vi "SaveDataSet.vi"(6 "AssetNodeMap":variant, 7 "do not write to database":bool, 8 "error in (no error)":errorcluster, 9 "Waveform":waveform(sgl), 10 "DataSetRegistry":T1, 11 "event in":T3) -> (0 "error out":errorcluster, 3 "event out":T3)   [LabVIEW 2017, in "CmsDataEventCreator.lvlib"]
uses:
  <vilib>/addons/InsightCM/Devices/Shared/Cms/CmsDataEventCreator/CmsDataEventCreator.lvlib
  <vilib>/addons/InsightCM/Devices/Shared/Common/DataEvent/controls/Event.ctl
  <vilib>/addons/InsightCM/MessageBus/Base/controls/DataEvent.ctl
  <vilib>/addons/InsightCM/MessageBus/Base/controls/KeyValuePair.ctl
  <vilib>/addons/InsightCM/Devices/Shared/Common/DataEvent/controls/DataSet.ctl
  <vilib>/addons/InsightCM/MessageBus/Base/controls/DataSetMetadata.ctl
  <vilib>/addons/InsightCM/MessageBus/Base/controls/TrendPoint.ctl
  <vilib>/addons/InsightCM/MessageBus/Base/controls/TrendAlarmUpdate.ctl
  <vilib>/addons/InsightCM/MessageBus/Base/controls/TrendAlarmTransition.ctl
  <vilib>/addons/InsightCM/Devices/Shared/Cms/CmsDataEventCreator/controls/DataSetRegistry.ctl
  <vilib>/addons/InsightCM/Devices/Shared/Common/DataEvent/controls/DataSetType.ctl
  <vilib>/addons/InsightCM/Devices/Shared/Common/DataEventCreator/DataEventCreator.lvlib
  <vilib>/addons/InsightCM/Utilities/PropertyHelpers/PropertyHelpers.lvlib
  <vilib>/addons/InsightCM/Devices/Shared/Common/DataEvent/DataEvent.lvlib
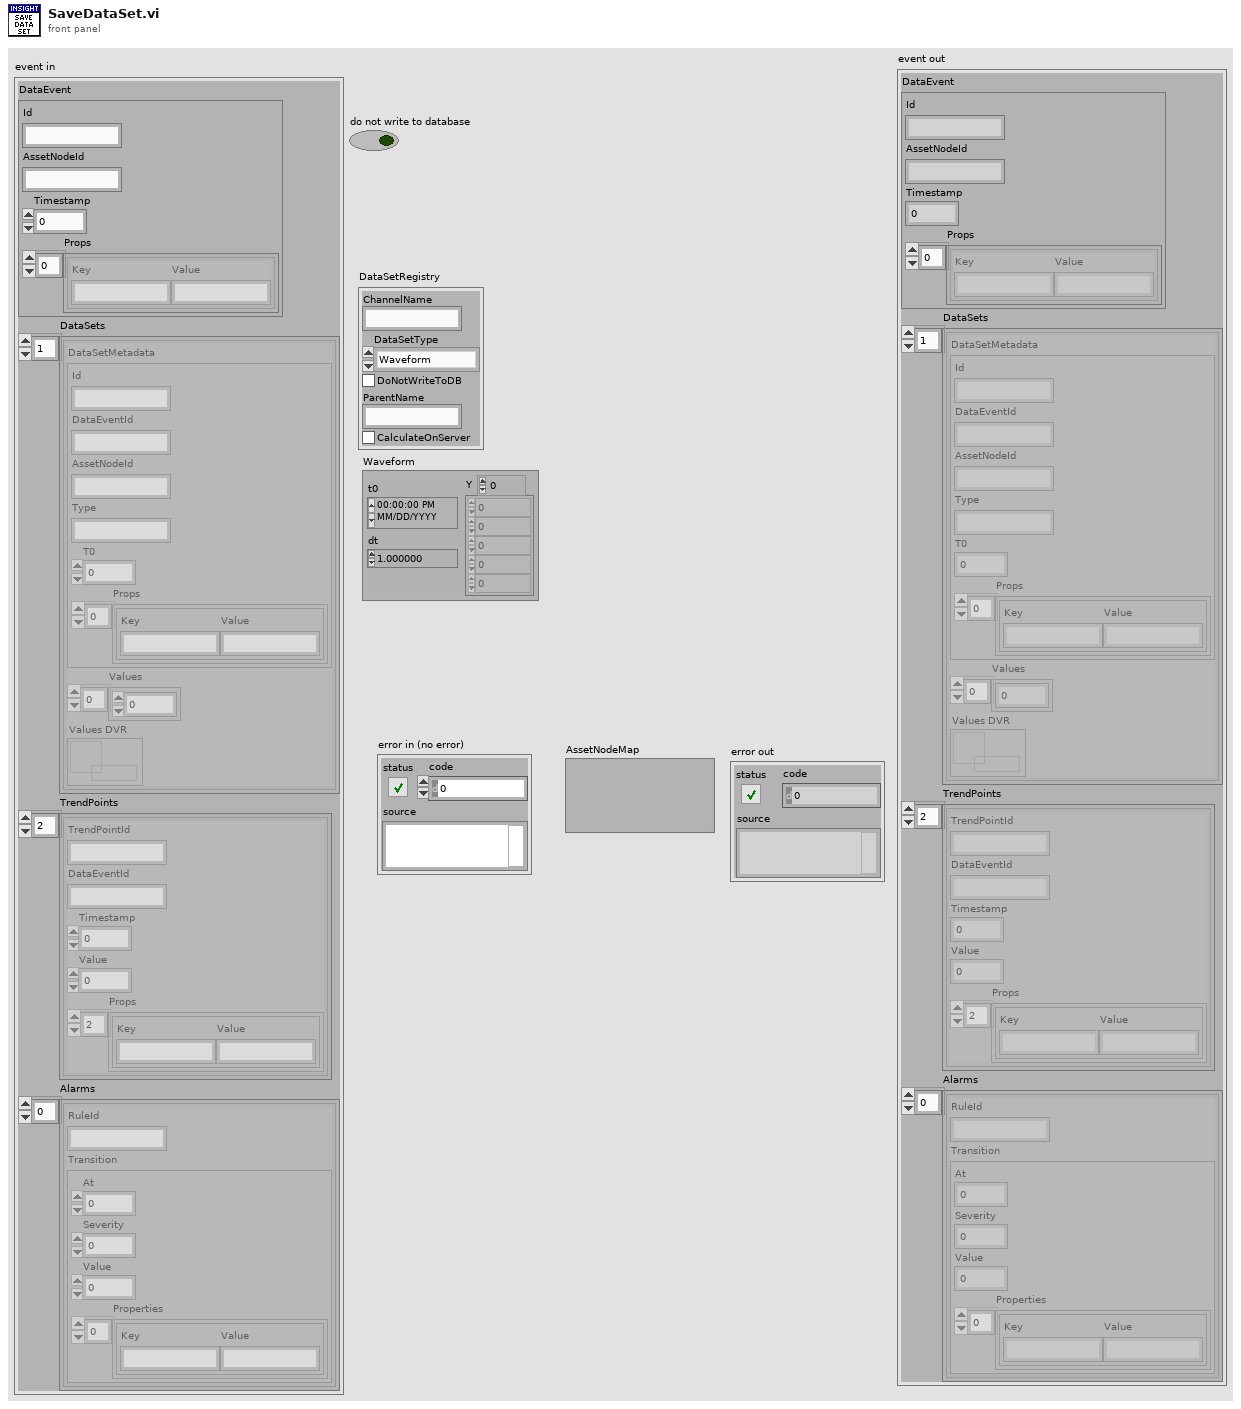
[diagram p1: front panel]
types:
  T1 = typedef "CmsDataEventCreator.lvlib/DataSetRegistry.ctl" = cluster{"ChannelName":string, "DataSetType":T2, "DoNotWriteToDB":bool, "ParentName":string, "CalculateOnServer":bool}
  T2 = typedef "DataEvent.lvlib/DataSetType.ctl" = enum16{"Waveform", "SpeedProfile", "ThermalImage", "EmsaSweep"}
  T3 = typedef "DataEvent.lvlib/Event.ctl" = cluster{"DataEvent":T4, "DataSets":T6[], "TrendPoints":T8[], "Alarms":T9[]}
  T4 = typedef "DataEvent.ctl" = cluster{"Id":string, "AssetNodeId":string, "Timestamp":i64, "Props":T5[]}
  T5 = typedef "KeyValuePair.ctl" = cluster{"Key":string, "Value":string}
  T6 = typedef "DataEvent.lvlib/DataSet.ctl" = cluster{"DataSetMetadata":T7, "Values":sgl[], "Values DVR":refnum<data-value>}
  T7 = typedef "DataSetMetadata.ctl" = cluster{"Id":string, "DataEventId":string, "AssetNodeId":string, "Type":string, "T0":i64, "Props":T5[]}
  T8 = typedef "TrendPoint.ctl" = cluster{"TrendPointId":string, "DataEventId":string, "Timestamp":i64, "Value":dbl, "Props":T5[]}
  T9 = typedef "TrendAlarmUpdate.ctl" = cluster{"RuleId":string, "Transition":T10}
  T10 = typedef "TrendAlarmTransition.ctl" = cluster{"At":i64, "Severity":i32, "Value":dbl, "Properties":T5[]}
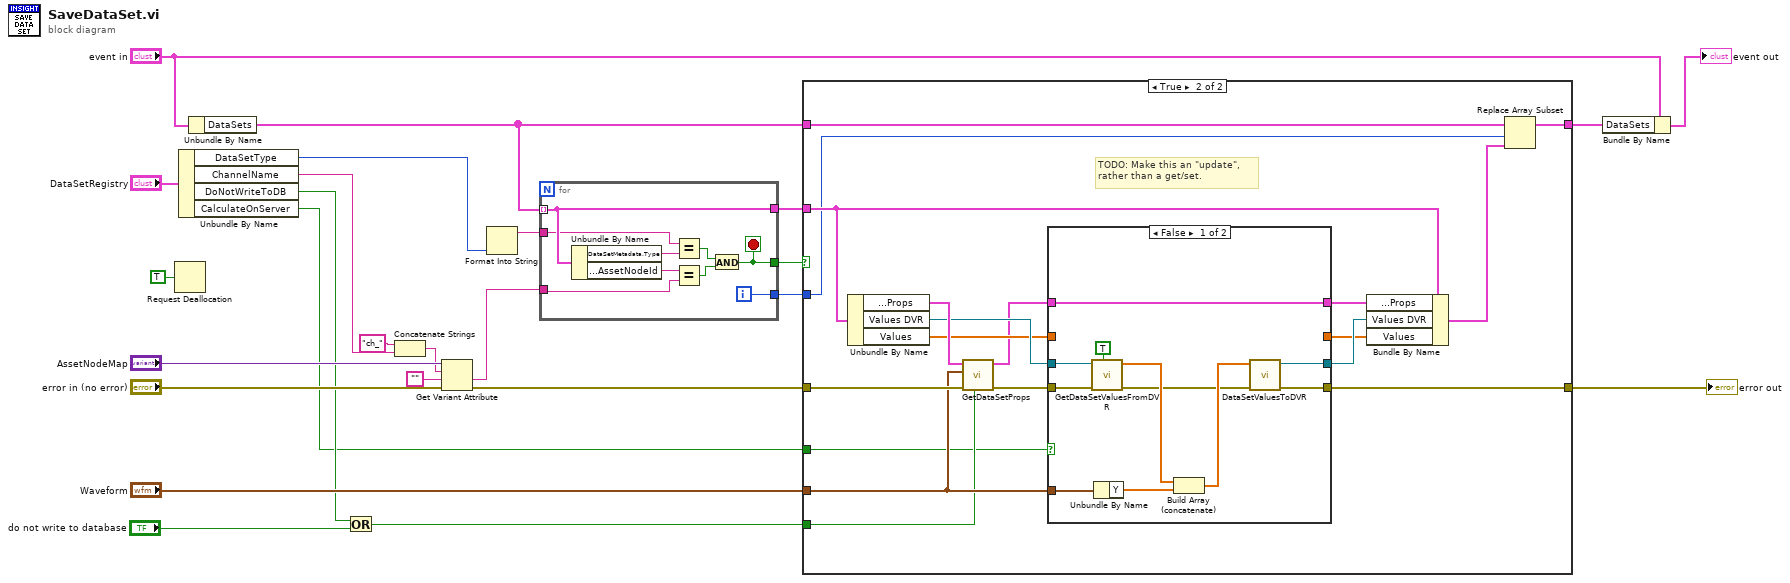
[diagram p0: block diagram]
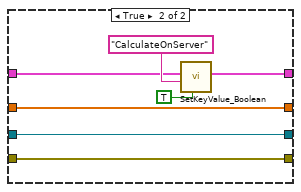
[diagram p3: hidden frame]
diagram:
  n1 = Request Deallocation(TRUE ("flag")) -> ()
  n2 = Unbundle By Name("DataSetRegistry") -> ("DataSetType"=w12:T2, "ChannelName"=w3:string, "DoNotWriteToDB"=w7:bool, "CalculateOnServer"=w5:bool)
  n3 = Unbundle By Name("event in") -> ("DataSets"=w19:T6[])
  n4 = Or(x=w7, y="do not write to database") -> (x .or. y?=w6:bool)
  n5 = Concatenate Strings("ch_" ("string"), w3) -> (w2:string)
  n6 = Get Variant Attribute(Variant="AssetNodeMap", name=w2, default value (empty Variant)="", error in="error in (no error)") -> (value=w21:string, error out=w10:errorcluster)  [unwired: 2 out]
  n7 = Format Into String(w12) -> (resulting string=w11:string)  [unwired: 3 in, 1 out]
  n8 = for {
    tunnel: w19 -> [w32] mode=indexing
    tunnel: w21 -> [w33]
    tunnel: [w28] -> w22
    tunnel: [w32] -> w16
    tunnel: [w31] -> w15
    tunnel: w11 -> [w26]
    i -> [w31]
    stop <- w28 stop-if-true
    n9 = Unbundle By Name(w32) -> ("DataSetMetadata.Type"=w27:string, "DataSetMetadata.AssetNodeId"=w34:string)
    n10 = Equal?(x=w26, y=w27) -> (x = y?=w30:bool)
    n11 = Equal?(x=w34, y=w33) -> (x = y?=w29:bool)
    n12 = And(x=w30, y=w29) -> (x .and. y?=w28:bool)
  }
  n13 = case shown="True" w22 {
    tunnel: w10 -> [w35 w49]
    tunnel: w19 -> [w36 w53]
    tunnel: [w36 w52] -> w18
    tunnel: w16 -> [_ w54]
    tunnel: w15 -> [_ w51]
    tunnel: [w35 w41] -> w13
    tunnel: "Waveform" -> [_ w48]
    tunnel: w6 -> [_ w46]
    tunnel: w5 -> [_ w45]
    frame False {
    }
    frame True {
      # "TODO: Make this an \"update\",\nrather than a get/set."
      n14 = Unbundle By Name(w54) -> ("DataSetMetadata.Props"=w47:T5[], "Values DVR"=w44:refnum<data-value>, "Values"=w40:sgl[])
      n15 = call <vilib>:"GetDataSetProps.vi"("do not write to database"=w46, "error in (no error)"=w49, "waveform"=w48, "dataset props in"=w47) -> ("error out"=w42:errorcluster, "dataset props out"=w37:T5[])  [unwired: 6 in]
      n16 = case shown="False" w45 {
        tunnel: w48 -> [w64 _]
        tunnel: w44 -> [w63 w72]
        tunnel: [w60 w72] -> w43
        tunnel: [w58 w71] -> w41
        tunnel: w42 -> [w57 w71]
        tunnel: w40 -> [_ w70]
        tunnel: [_ w70] -> w39
        tunnel: [w55 w67] -> w38
        tunnel: w37 -> [w55 w66]
        frame False {
          n17 = call <vilib>:"GetDataSetValuesFromDVR.vi"("delete dvr"=TRUE, "error in (no error)"=w57, "values dvr"=w63) -> ("error out"=w59:errorcluster, "values"=w62:sgl[])  [unwired: 7 in]
          n18 = Unbundle By Name(w64) -> ("Y"=w65:sgl[])
          n19 = Build Array (concatenate)(w62, w65) -> (w61:sgl[])
          n20 = call <vilib>:"DataSetValuesToDVR.vi"("error in (no error)"=w59, "dataset values"=w61) -> ("error out"=w58:errorcluster, "new dataset values dvr"=w60:refnum<data-value>)  [unwired: 8 in]
        }
        frame True {
          n21 = call <vilib>:"SetKeyValue_Boolean.vi"("value"=TRUE, "key"="CalculateOnServer", "key value pairs"=w66) -> ("key value pairs out"=w67:T5[])  [unwired: 8 in]
        }
      }
      n22 = Bundle By Name(cluster=w54, "DataSetMetadata.Props"=w38, "Values DVR"=w43, "Values"=w39) -> (w50:T6)
      n23 = Replace Array Subset(array=w53, new element=w50, index=w51) -> (w52:T6[])
    }
  }
  "error out" <- w13
  n24 = Bundle By Name(cluster="event in", "DataSets"=w18) -> (→"event out":T3)
